vi "CryptReleaseContext.vi"(8 "error in (no error)":errorcluster, 11 "CSP handle in":u32) -> (0 "error out":errorcluster, 4 "operation status":string)   [LabVIEW 2013]
doc: "Releases the handle of a cryptographic service provider (CSP) and a key container.\n\nhttps://msdn.microsoft.com/pl-pl/library/windows/desktop/aa380268(v=vs.85).aspx"
uses:
  advapi32.dll
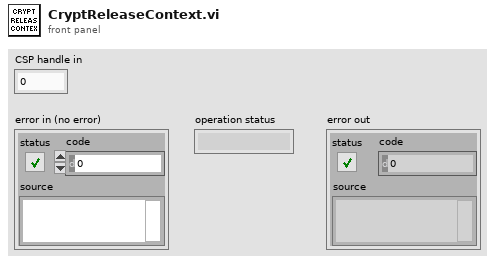
[diagram p1: front panel]
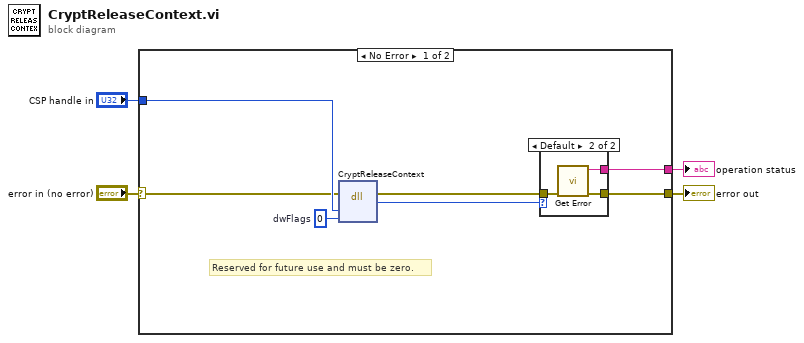
[diagram p0: block diagram]
diagram:
  n1 = case shown="No Error" "error in (no error)" {
    selector: "error in (no error)" -> [w5 w16]
    tunnel: "CSP handle in" -> [w10 _]
    tunnel: [w7 _] -> w3
    tunnel: [w6 w16] -> w2
    frame No Error {
      w11 = u32 0  # dwFlags
      # "Reserved for future use and must be zero."
      n2 = dll-call lib="advapi32.dll" fn="CryptReleaseContext"(error in=w5, "hProv"=w10, "dwFlags"=w11) -> (error out=w8:errorcluster, "return type"=w9:i32)  [unwired: 4 in, 1 out]
      n3 = case shown="Default" w9 {
        tunnel: [w12 w15] -> w6
        tunnel: [_ w14] -> w7
        tunnel: w8 -> [w12 w13]
        frame 0 {
        }
        frame Default {
          n4 = call "Get Error.vi"("error in (no error)"=w13) -> ("error out"=w15:errorcluster, "lpBuffer"=w14:string)  [unwired: 9 in]
        }
      }
    }
    frame Error {
    }
  }
  "error out" <- w2
  "operation status" <- w3
